vi "CSM - Global Log Monitoring Loop.vi"() -> ()   [LabVIEW 2017, in "CSM-QuickDrops.lvlib"]
uses:
  CSM-QuickDrops.lvlib
  _Support/Typedef/_CSM_GlobalLog_MSG.ctl
  _Support/Typedef/_CSM_Response Source Message.ctl
  _Support/Typedef/_CSM_GlobalLog_MSG_TYPE.ctl
  <vilib>/Utility/error.llb/Clear Errors.vi
  _Support/GlobalEvent/Gevt-ThreadQueueName.vi
  _Support/FGV-BroadcastRegistry/global-CSMQ FGV Change Flag.vi
  _Support/CSMQ/_CSMOFGV.vi
  Communicable State Machine.lvlib
panel:
  out "State History":string
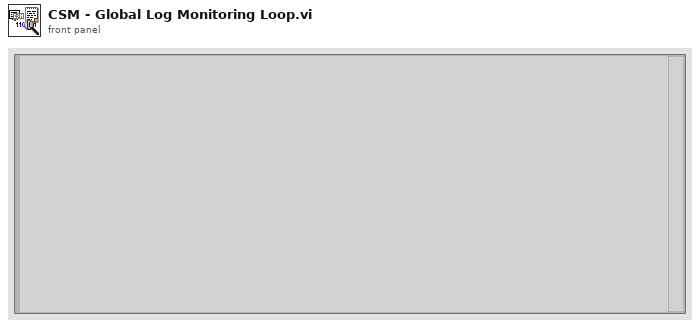
[diagram p1: front panel]
types:
  T1 = cluster{"threashold(#/s)":dbl, "Check Peroid(s)":dbl}
  T2 = typedef "Communicable State Machine.lvlib/_CSM_GlobalLog_MSG.ctl" = cluster{"Name(\"\" to use uuid)":string, "Current State":string, "Arguments":string, "Source Message":T3, "Source Module":string, "Complete(T)/Start(F)":bool, "LogType":T4}
  T3 = typedef "Communicable State Machine.lvlib/_CSM_Response Source Message.ctl" = cluster{"‘State":string, "’Arguments":string, "’Error":errorcluster}
  T4 = typedef "Communicable State Machine.lvlib/_CSM_GlobalLog_MSG_TYPE.ctl" = enum16{"User Log", "State Change", "Status", "Interrupt", "Register", "Unregister", "Error Log", "Module Created", "Module Destroyed"}
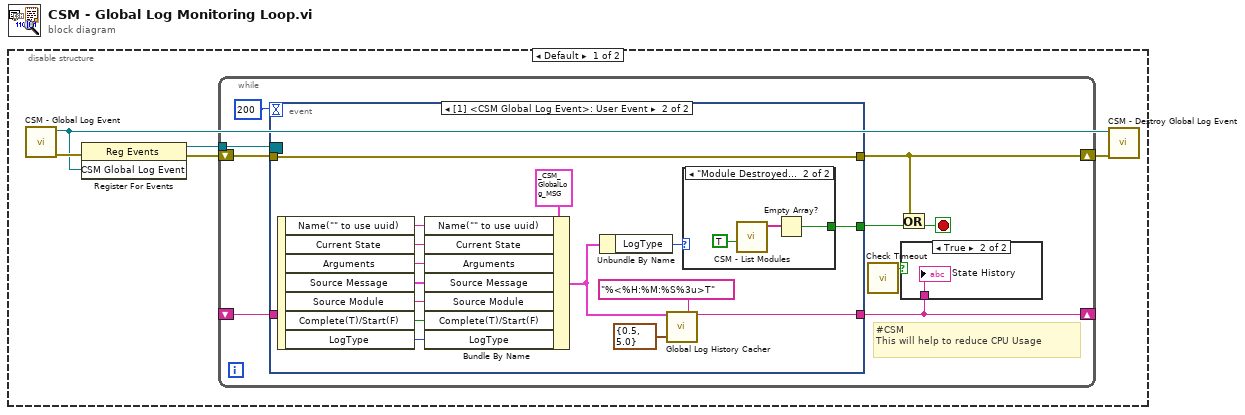
[diagram p0: block diagram]
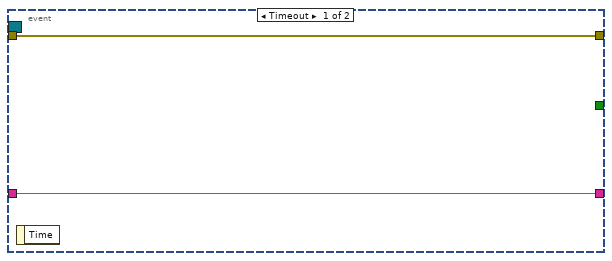
[diagram p3: hidden frame]
diagram:
  n1 = disable-structure shown="Default" {
    frame condition #0 (active) {
      n2 = call "CSM - Global Log Event.vi"() -> ("Error out"=w3:errorcluster, "CSM Global Log Event"=w1:refnum<user-event>)  [unwired: 10 in]
      n3 = register-events(error in=w3, w1) -> (reference out=w4:refnum<event-registration>, error out=w5:errorcluster)  [unwired: 1 in]
      n4 = while {
        tunnel: w4 -> [w14]
        shift-right: [w11] -> w2
        shift-left: w5 -> [w13]
        shift-right: [w8] -> _
        shift-left: _ -> [w7]
        stop <- w12 stop-if-true
        # "#CSM\nThis will help to reduce CPU Usage"
        n5 = event shown="[1] <CSM Global Log Event>: User Event" {
          selector: w14 -> [_ _]
          dyn-events: _ -> [_ _]
          timeout: 200 -> [_ _]
          tunnel: w13 -> [w17 w32]
          tunnel: [w17 w32] -> w11
          tunnel: [_ w21] -> w10
          tunnel: [w16 w18] -> w8
          tunnel: w7 -> [w16 _]
          event Timeout {
            n6 = event-data() -> ()  [unwired: 1 in, 1 out]
          }
          event User Event {
            n7 = event-data() -> ("Name(\"\" to use uuid)"=w31:string, "Current State"=w30:string, "Arguments"=w29:string, "Source Message"=w28:T3, "Source Module"=w27:string, "Complete(T)/Start(F)"=w26:bool, "LogType"=w25:T4)  [unwired: 1 in]
            n8 = Bundle By Name(cluster=T2 {"Name(\"\" to use uuid)"="", "Current State"="", "Arguments"="", "Source Message"={"‘State"="", "’Arguments"="", "’Error"={"status"=FALSE, "code"=0, "source"=""}}, "Source Module"="", "Complete(T)/Start(F)"=FALSE, "LogType"=enum."State Change"} ("Cross CSM Data"), "Name(\"\" to use uuid)"=w31, "Current State"=w30, "Arguments"=w29, "Source Message"=w28, "Source Module"=w27, "Complete(T)/Start(F)"=w26, "LogType"=w25) -> (w23:T2)
            n9 = Unbundle By Name(w23) -> ("LogType"=w22:T4)
            n10 = call "Global Log History Cacher.vi"("Cross CSM Data"=w23, "Time format string"="%<%H:%M:%S%3u>T", "Settings"=T1 {"threashold(#/s)"=0.5, "Check Peroid(s)"=5.0}) -> ("String Cache"=w18:string)  [unwired: 11 in, 1 out]
            n11 = case shown="\"Module Destroyed\"" w22 {
              tunnel: [_ w33] -> w21
              frame "User Log", Default {
              }
              frame "Module Destroyed" {
                n12 = call "CSM - List Modules.vi"("All?"=TRUE) -> ("Module Names"=w35:string[])  [unwired: 9 in, 1 out]
                n13 = Empty Array?(array=w35) -> (empty?=w33:bool)
              }
            }
          }
        }
        n14 = call "Check Timeout.vi"() -> ("Timeout"=w6:bool)  [unwired: 8 in]
        n15 = Or(x=w11, y=w10) -> (x .or. y?=w12:bool)
        n16 = case shown="True" w6 {
          tunnel: w8 -> [_ w15]
          frame False {
          }
          frame True {
            "State History" <- w15
          }
        }
      }
      n17 = call "CSM - Destroy Global Log Event.vi"("Error in"=w2, "CSM Global Log Event"=w1) -> ()  [unwired: 9 in, 1 out]
    }
    frame condition #1 {
    }
  }
